vi "FL Get Membership Function (Fuzzy System).vi"(0 "fuzzy system in":T3 {"user MF interpolating polynomials"."coa_x(y) coeff" format="%.4g"; "user MF interpolating polynomials"."Area(y) coeff" format="%.4g"; "user MF interpolating polynomials"."X(y) coeff" format="%.4g"; "user MF interpolating polynomials"."Y(x) coeff" format="%.4g"; "user MF interpolating polynomials"."Y" format="%.4g"; "user MF interpolating polynomials"."X" format="%.4g"; "defuzzification method" items=["Center of Area", "Modified Center of Area", "Center of Sums", "Center of Maximum", "Mean of Maximum"]; "rules"."consequents"."Var Index" min=0; "rules"."consequents"."Cond" items=["=", "!="]; "rules"."consequents"."MF Index" min=0; "rules"."antecedents"."Var Index" min=0; "rules"."antecedents"."Cond" items=["=", "!="]; "rules"."antecedents"."MF Index" min=0; "rules"."consequent implication" items=["Minimum", "Product"]; "rules"."antecedent connective" items=["AND (Minimum)", "AND (Product)", "OR (Maximum)", "OR (Probabilistic)"]; "output variables"."MFs"."shape" items=["Triangle", "Trapezoid", "Singleton", "Sigmoid", "Gaussian", "User-Defined"]; "input variables"."MFs"."shape" items=["Triangle", "Trapezoid", "Singleton", "Sigmoid", "Gaussian", "User-Defined"]}, 1 "input/output":T1 items=["Input", "Output"], 2 "variable index":i32, 3 "membership function index":i32, 11 "error in (no error)":errorcluster) -> (4 "fuzzy system out":T3 {"user MF interpolating polynomials"."coa_x(y) coeff" format="%.4g"; "user MF interpolating polynomials"."Area(y) coeff" format="%.4g"; "user MF interpolating polynomials"."X(y) coeff" format="%.4g"; "user MF interpolating polynomials"."Y(x) coeff" format="%.4g"; "user MF interpolating polynomials"."Y" format="%.4g"; "user MF interpolating polynomials"."X" format="%.4g"; "defuzzification method" items=["Center of Area", "Modified Center of Area", "Center of Sums", "Center of Maximum", "Mean of Maximum"]; "rules"."consequents"."Var Index" min=0; "rules"."consequents"."Cond" items=["=", "!="]; "rules"."consequents"."MF Index" min=0; "rules"."antecedents"."Var Index" min=0; "rules"."antecedents"."Cond" items=["=", "!="]; "rules"."antecedents"."MF Index" min=0; "rules"."consequent implication" items=["Minimum", "Product"]; "rules"."antecedent connective" items=["AND (Minimum)", "AND (Product)", "OR (Maximum)", "OR (Probabilistic)"]; "output variables"."MFs"."shape" items=["Triangle", "Trapezoid", "Singleton", "Sigmoid", "Gaussian", "User-Defined"]; "input variables"."MFs"."shape" items=["Triangle", "Trapezoid", "Singleton", "Sigmoid", "Gaussian", "User-Defined"]}, 6 "name":string, 8 "shape":T2 items=["Triangle", "Trapezoid", "Singleton", "Sigmoid", "Gaussian", "User-Defined"], 10 "points":dbl[](array[numeric]), 13 "user-defined shape index":i32, 14 "color":u32(colorbox), 15 "error out":errorcluster)   [LabVIEW 2017, in "NI_Fuzzy_Logic_API.lvlib"]
doc: "Returns the shape, color, and points of a membership function for a linguistic variable. You can return a membership function from a fuzzy system or from an array of membership functions. The data type you wire to the <B>fuzzy system in</B> input determines the polymorphic instance to use."
uses:
  <vilib>/addons/Fuzzy Logic/NI_Fuzzy_Logic_API.lvlib
  <vilib>/addons/Fuzzy Logic/TypeDefs/FL System.ctl
  <vilib>/addons/Fuzzy Logic/TypeDefs/FL Variable.ctl
  <vilib>/addons/Fuzzy Logic/TypeDefs/FL Membership Function.ctl
  <vilib>/addons/Fuzzy Logic/TypeDefs/FL Membership Function Shape.ctl
  <vilib>/addons/Fuzzy Logic/TypeDefs/FL Rule.ctl
  <vilib>/addons/Fuzzy Logic/TypeDefs/FL Antecedent.ctl
  <vilib>/addons/Fuzzy Logic/TypeDefs/FL Modifier.ctl
  <vilib>/addons/Fuzzy Logic/TypeDefs/FL Antecedent Connective.ctl
  <vilib>/addons/Fuzzy Logic/TypeDefs/FL Consequent.ctl
  <vilib>/addons/Fuzzy Logic/TypeDefs/FL Consequent Implication.ctl
  <vilib>/addons/Fuzzy Logic/TypeDefs/FL Defuzzification.ctl
  <vilib>/addons/Fuzzy Logic/TypeDefs/FL Interpolating polynomials.ctl
  <vilib>/addons/Fuzzy Logic/TypeDefs/FL Input_Output.ctl
panel:
  # "IF"
  # "THEN"
  # "IF"
  # "THEN"
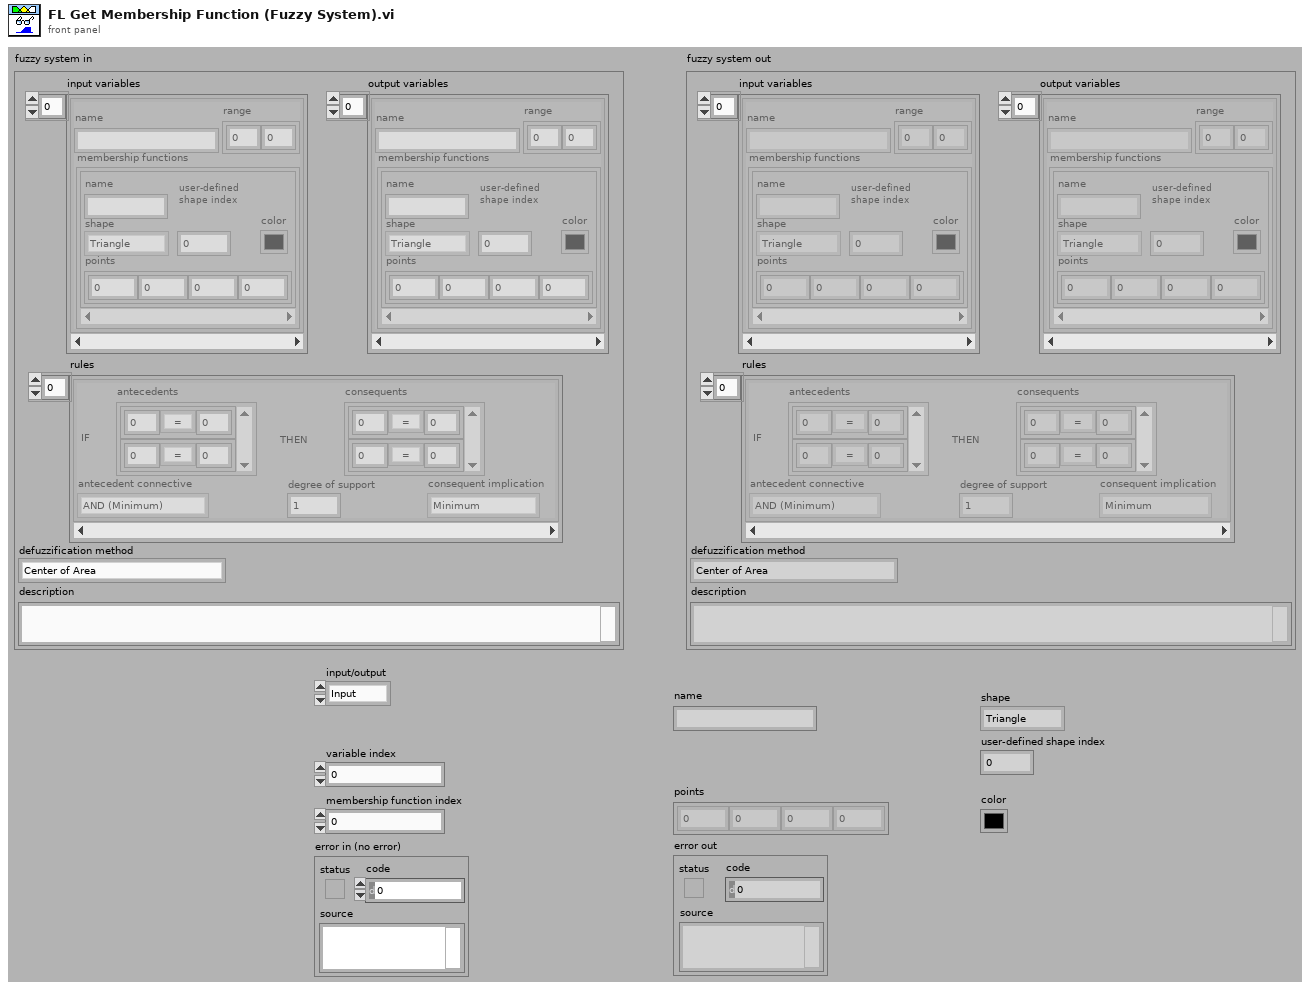
[diagram p1: front panel]
types:
  T1 = typedef "NI_Fuzzy_Logic_API.lvlib/FL Input_Output.ctl" = u16
  T2 = typedef "NI_Fuzzy_Logic_API.lvlib/FL Membership Function Shape.ctl" = u16
  T3 = typedef "NI_Fuzzy_Logic_API.lvlib/FL System.ctl" = cluster{"input variables":T4[], "output variables":T4[], "rules":T6[], "defuzzification method":T12, "description":string, "user MF interpolating polynomials":T13[]}
  T4 = typedef "NI_Fuzzy_Logic_API.lvlib/FL Variable.ctl" = cluster{"name":string, "range":dbl[], "MFs":T5[]}
  T5 = typedef "NI_Fuzzy_Logic_API.lvlib/FL Membership Function.ctl" = cluster{"name":string, "shape":T2, "points":dbl[], "color":u32, "user-defined shape index":i32}
  T6 = typedef "NI_Fuzzy_Logic_API.lvlib/FL Rule.ctl" = cluster{"antecedents":T7[], "antecedent connective":T9, "consequents":T10[], "consequent implication":T11, "degree of support":dbl}
  T7 = typedef "NI_Fuzzy_Logic_API.lvlib/FL Antecedent.ctl" = cluster{"Var Index":i32, "MF Index":i32, "Cond":T8}
  T8 = typedef "NI_Fuzzy_Logic_API.lvlib/FL Modifier.ctl" = u16
  T9 = typedef "NI_Fuzzy_Logic_API.lvlib/FL Antecedent Connective.ctl" = u16
  T10 = typedef "NI_Fuzzy_Logic_API.lvlib/FL Consequent.ctl" = cluster{"Var Index":i32, "MF Index":i32, "Cond":T8}
  T11 = typedef "NI_Fuzzy_Logic_API.lvlib/FL Consequent Implication.ctl" = u16
  T12 = typedef "NI_Fuzzy_Logic_API.lvlib/FL Defuzzification.ctl" = u16
  T13 = typedef "NI_Fuzzy_Logic_API.lvlib/FL Interpolating polynomials.ctl" = cluster{"X":dbl[], "Y":dbl[], "Y(x) coeff":dbl[][], "X(y) coeff":dbl[][], "Area(y) coeff":dbl[][], "coa_x(y) coeff":dbl[][]}
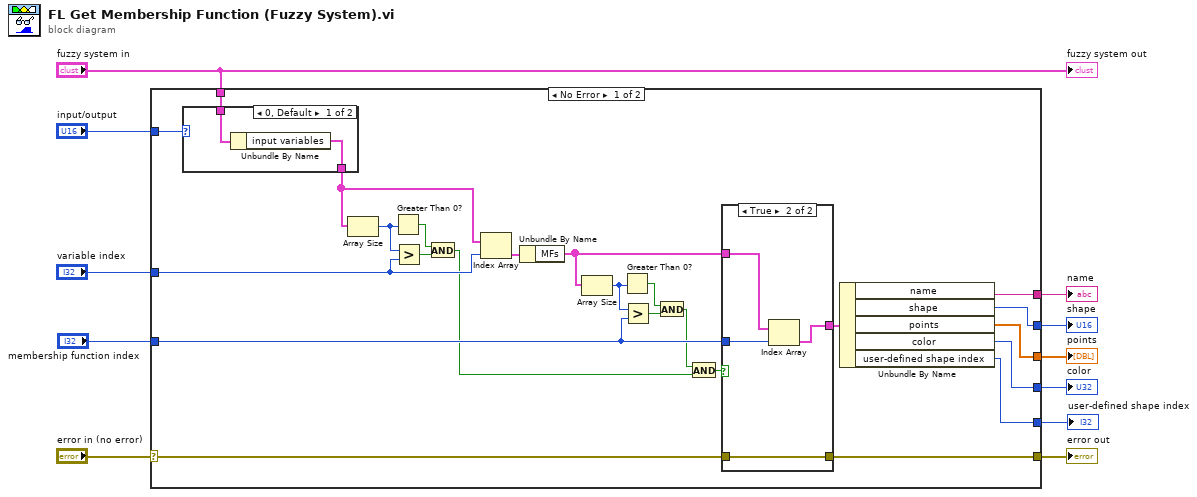
[diagram p0: block diagram]
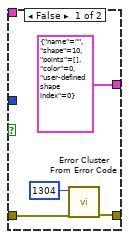
[diagram p2: hidden frame]
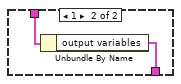
[diagram p3: hidden frame]
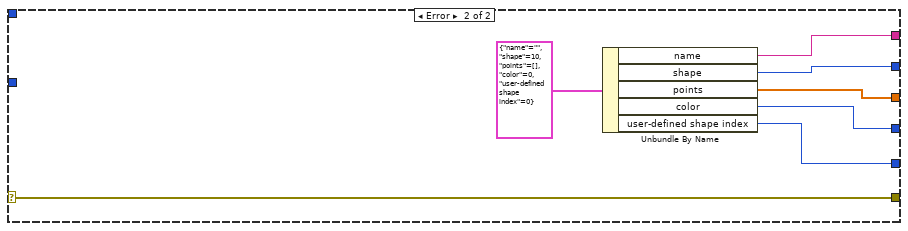
[diagram p4: hidden frame]
diagram:
  n1 = case shown="No Error" "error in (no error)" {
    selector: "error in (no error)" -> [w15 w54]
    tunnel: "membership function index" -> [w18 _]
    tunnel: "variable index" -> [w23 _]
    tunnel: "fuzzy system in" -> [w34 _]
    tunnel: [w31 w53] -> w8
    tunnel: [w29 w50] -> w7
    tunnel: [w28 w49] -> w6
    tunnel: [w30 w52] -> w5
    tunnel: "input/output" -> [w33 _]
    tunnel: [w14 w54] -> w2
    tunnel: [w12 w48] -> w1
    frame No Error {
      n2 = case shown="0, Default" w33 {
        tunnel: [w45 w46] -> w24
        tunnel: w34 -> [w44 w47]
        frame 0, Default {
          n3 = Unbundle By Name(w44) -> ("input variables"=w45:T4[])
        }
        frame 1 {
          n4 = Unbundle By Name(w47) -> ("output variables"=w46:T4[])
        }
      }
      n5 = Array Size(array=w24) -> (size(s)=w26:i32)
      n6 = Greater Than 0?(x=w26) -> (x > 0?=w27:bool)
      n7 = Greater?(x=w26, y=w23) -> (0:w25:bool)
      n8 = And(x=w27, y=w25) -> (x .and. y?=w16:bool)
      n9 = Index Array(array=w24, index=w23) -> (element=w35:T4)
      n10 = Unbundle By Name(w35) -> ("MFs"=w19:T5[])
      n11 = Array Size(array=w19) -> (size(s)=w21:i32)
      n12 = Greater Than 0?(x=w21) -> (x > 0?=w20:bool)
      n13 = Greater?(x=w21, y=w18) -> (0:w22:bool)
      n14 = And(x=w20, y=w22) -> (x .and. y?=w17:bool)
      n15 = And(x=w17, y=w16) -> (x .and. y?=w13:bool)
      n16 = case shown="True" w13 {
        tunnel: [T5 {"name"="", "shape"=10, "points"=[], "color"=0, "user-defined shape index"=0} ("MF") w43] -> w32
        tunnel: w19 -> [_ w42]
        tunnel: w18 -> [_ w41]
        tunnel: w15 -> [w37 w40]
        tunnel: [w38 w40] -> w14
        frame False {
          n17 = call <vilib>:"Error Cluster From Error Code.vi"("error in (no error)"=w37, "error code (0)"=1304) -> ("error out"=w38:errorcluster)  [unwired: 1 in, 6 out]
        }
        frame True {
          n18 = Index Array(array=w42, index=w41) -> (element=w43:T5)
        }
      }
      n19 = Unbundle By Name(w32) -> ("name"=w31:string, "shape"=w30:T2, "points"=w29:dbl[], "color"=w28:u32, "user-defined shape index"=w12:i32)
    }
    frame Error {
      n20 = Unbundle By Name(T5 {"name"="", "shape"=10, "points"=[], "color"=0, "user-defined shape index"=0} ("MF")) -> ("name"=w53:string, "shape"=w52:T2, "points"=w50:dbl[], "color"=w49:u32, "user-defined shape index"=w48:i32)
    }
  }
  "name" <- w8
  "points" <- w7
  "color" <- w6
  "shape" <- w5
  "error out" <- w2
  "user-defined shape index" <- w1
  "fuzzy system out" <- "fuzzy system in"
